vi "Gain.vi"() -> ()   [LabVIEW 2010]
panel:
  in  "Gain":u32
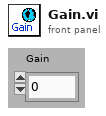
[diagram p1: front panel]
diagram:
